vi "Write UART.vi"(7 "UART":u8, 8 "error in (no error)":errorcluster, 10 "Data":string, 11 "VISA resource name in":refnum<visa-resource-name>) -> (0 "error out":errorcluster, 3 "VISA resource name":refnum<visa-resource-name>)   [LabVIEW 2024, in "CTIPicoVISA.lvlib"]
uses:
  CTIPicoVISA.lvlib
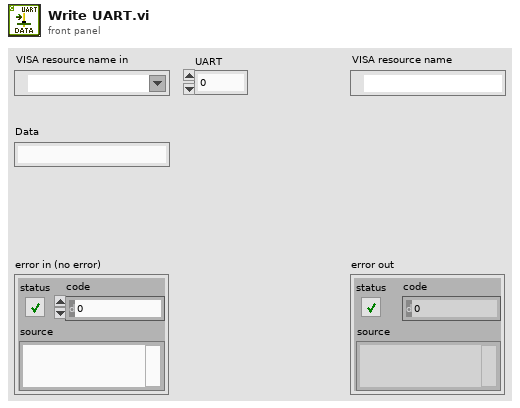
[diagram p1: front panel]
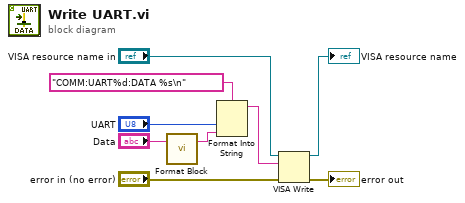
[diagram p0: block diagram]
diagram:
  n1 = call "Format Block.vi"("Data Block"="Data") -> ("Formatted Block"=w1:string)  [unwired: 6 in]
  n2 = Format Into String(format string="COMM:UART%d:DATA %s\n", "UART", w1) -> (resulting string=w5:string)  [unwired: 2 in, 1 out]
  n3 = VISA Write(VISA resource name="VISA resource name in", write buffer=w5, error in (no error)="error in (no error)") -> (VISA resource name out=→"VISA resource name":refnum<visa-resource-name>, error out=→"error out":errorcluster)  [unwired: 1 out]
